vi "Init Notebook Rich Text Box.vi"(8 "Error In":errorcluster, 9 "Notebook Content":string, 11 ".NET Refnum in":refnum<k24>) -> (0 "Error Out":errorcluster)   [LabVIEW 2021, in "Notebook.lvlib"]
uses:
  Notebook.lvlib
  System.Windows.Forms
  System.Drawing
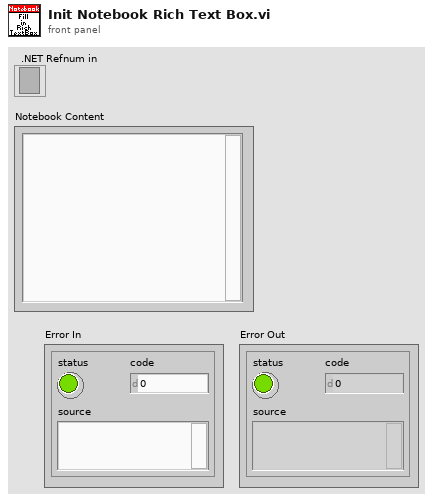
[diagram p1: front panel]
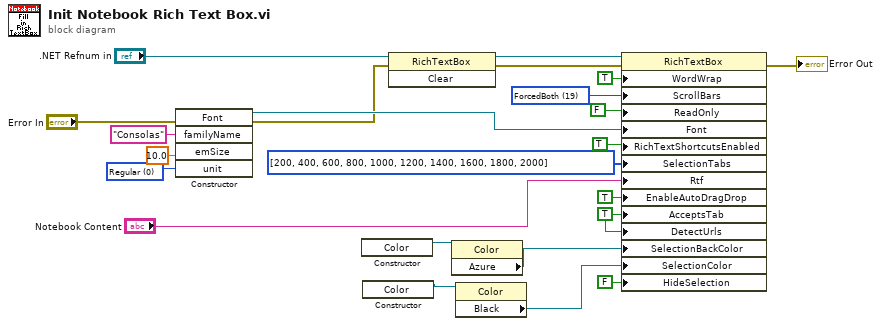
[diagram p0: block diagram]
diagram:
  w6 = TRUE ("ContainsFocus")
  w21 = 0 items=["Regular"=0, "Bold"=1, "Italic"=2, "Underline"=4, "Strikeout"=8] ("style")
  w12 = 19 items=["None"=0, "Horizontal"=1, "Vertical"=2, "Both"=3, "ForcedHorizontal"=17, "ForcedVertical"=18, "ForcedBoth"=19] ("ScrollBars")
  n1 = constructor class="Font"(error in="Error In", "familyName"="Consolas", "emSize"=sgl 10.0, "unit"=w21) -> (reference out=w23:refnum<k24>, error out=w15:errorcluster)  [unwired: 2 in, 4 out]
  n2 = constructor class="Color"() -> (reference out=w5:refnum<k24>)  [unwired: 3 in, 2 out]
  n3 = constructor class="Color"() -> (reference out=w3:refnum<k24>)  [unwired: 3 in, 2 out]
  n4 = invoke class="RichTextBox" method="Clear"(reference=".NET Refnum in", error in=w15) -> (reference out=w14:refnum<k24>, error out=w13:errorcluster)  [unwired: 1 in, 1 out]
  n5 = property class="Color"(reference=w5) -> ("Azure"=w4:refnum<k24>)  [unwired: 1 in, 2 out]
  n6 = property class="Color"(reference=w3) -> ("Black"=w2:refnum<k24>)  [unwired: 1 in, 2 out]
  n7 = property class="RichTextBox"(reference=w14, error in=w13, "WordWrap"=TRUE, "ScrollBars"=w12, "ReadOnly"=FALSE ("Enabled"), "Font"=w23, "RichTextShortcutsEnabled"=TRUE, "SelectionTabs"=i32[] [200, 400, 600, 800, 1000, 1200, 1400, 1600, 1800, 2000], "Rtf"="Notebook Content", "EnableAutoDragDrop"=TRUE, "AcceptsTab"=w6, "DetectUrls"=w6, "SelectionBackColor"=w4, "SelectionColor"=w2, "HideSelection"=FALSE) -> (error out=→"Error Out":errorcluster)  [unwired: 1 out]
